vi "VICI_unified.vi"(11 "RequestedValve#":i32) -> ()   [LabVIEW 2019]
panel:
  out "VICI 2 Error":bool
  out "VICI2 Read Position":i32
  out "VICI1 Error":bool
  out "VICI1 Read Position":i32
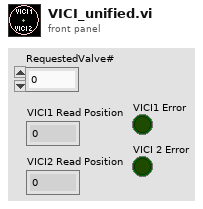
[diagram p1: front panel]
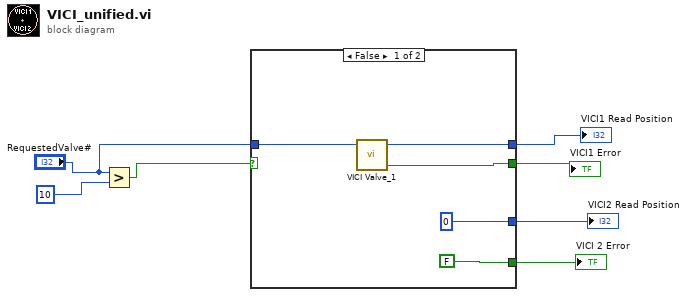
[diagram p0: block diagram]
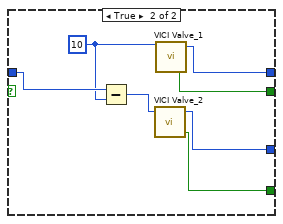
[diagram p2: hidden frame]
diagram:
  n1 = Greater?(x="RequestedValve#", y=10) -> (0:w7:bool)
  n2 = case shown="False" w7 {
    tunnel: "RequestedValve#" -> [w12 w19]
    tunnel: [w11 w16] -> w4
    tunnel: [w10 w15] -> w3
    tunnel: [0 ("Read Position") w14] -> w2
    tunnel: [FALSE ("Error? (bool)") w13] -> w1
    frame False {
      n3 = call "VICI Valve_1.vi"("RequestedValve#"=w12) -> ("Error? (bool)"=w10:bool, "Read Position"=w11:i32)  [unwired: 2 in, 1 out]
    }
    frame True {
      w18 = 10 ("y")
      n4 = Subtract(x=w19, y=w18) -> (x-y=w17:i32)
      n5 = call "VICI Valve_2.vi"("RequestedValve#"=w17) -> ("Error? (bool)"=w13:bool, "Read Position"=w14:i32)  [unwired: 2 in, 1 out]
      n6 = call "VICI Valve_1.vi"("RequestedValve#"=w18) -> ("Error? (bool)"=w15:bool, "Read Position"=w16:i32)  [unwired: 2 in, 1 out]
    }
  }
  "VICI1 Read Position" <- w4
  "VICI1 Error" <- w3
  "VICI2 Read Position" <- w2
  "VICI 2 Error" <- w1
